vi "Get Recursive Dependency List.vi"(8 "error in":errorcluster, 11 "dependency paths":path[](array[path])) -> (0 "error out":errorcluster, 2 "instr containing":path[](array[path]), 3 "array":path[](array[path]))   [LabVIEW 2021, in "Converter.lvlib"]
uses:
  Converter.lvlib
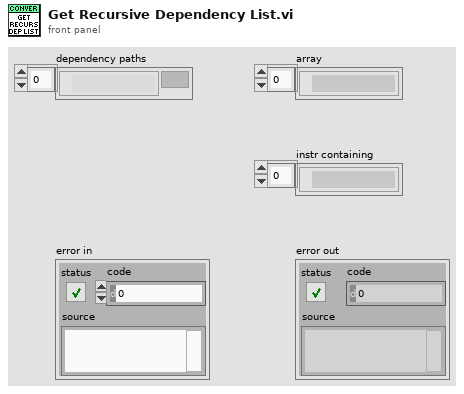
[diagram p1: front panel]
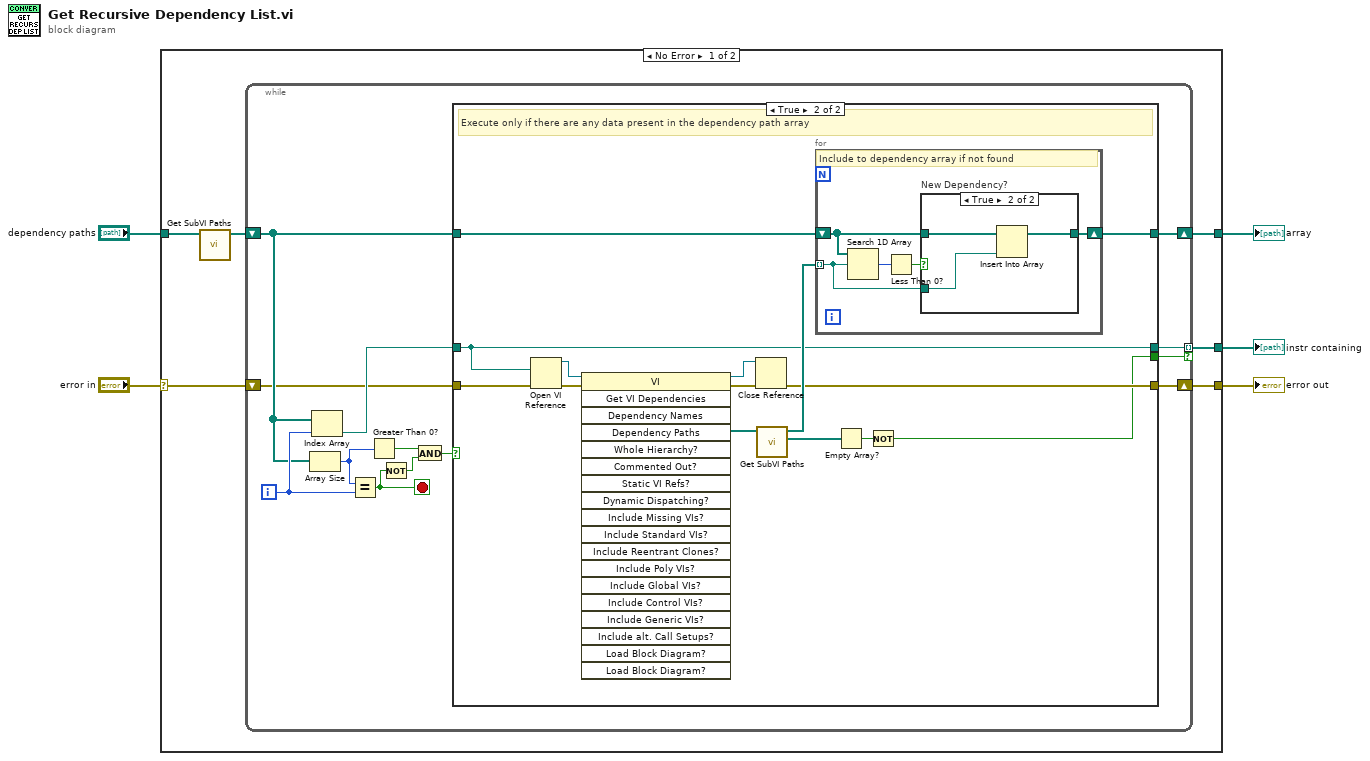
[diagram p0: block diagram]
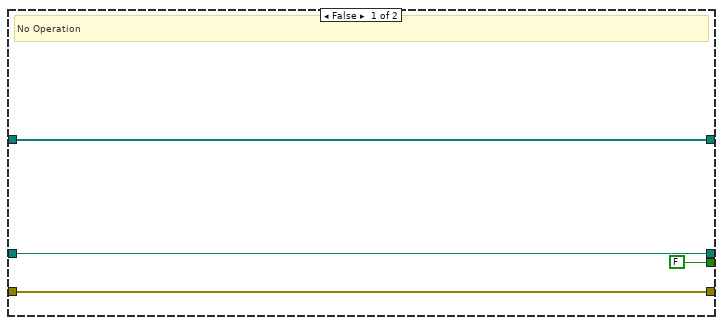
[diagram p2: hidden frame]
diagram:
  n1 = case shown="No Error" "error in" {
    selector: "error in" -> [w10 w52]
    tunnel: [w11 w52] -> w5
    tunnel: [w9 _] -> w3
    tunnel: "dependency paths" -> [w7 _]
    tunnel: [w6 _] -> w1
    frame No Error {
      n2 = call "Get SubVI Paths.vi"("dependency paths"=w7) -> ("actual dependencies[]"=w8:path[])  [unwired: 9 in, 1 out]
      n3 = while {
        shift-right: [w22] -> w9
        shift-left: w8 -> [w23]
        shift-right: [w19] -> w11
        shift-left: w10 -> [w20]
        tunnel: [w13] -> w6 mode=indexing if=w12
        i -> [w24]
        stop <- w17 stop-if-true
        n4 = Array Size(array=w23) -> (size(s)=w18:i32)
        n5 = Index Array(array=w23, index=w24) -> (element=w21:path)
        n6 = Equal?(x=w18, y=w24) -> (x = y?=w17:bool)
        n7 = Greater Than 0?(x=w18) -> (x > 0?=w15:bool)
        n8 = Not(x=w17) -> (.not. x?=w14:bool)
        n9 = And(x=w15, y=w14) -> (x .and. y?=w16:bool)
        n10 = case shown="True" w16 {
          tunnel: w23 -> [w27 w38]
          tunnel: [w27 w37] -> w22
          tunnel: w21 -> [w26 w32]
          tunnel: w20 -> [w28 w36]
          tunnel: [w28 w35] -> w19
          tunnel: [w26 w32] -> w13
          tunnel: [FALSE w31] -> w12
          frame False {
            # "No Operation"
          }
          frame True {
            # "Execute only if there are any data present in the dependency path array"
            n11 = Open VI Reference(vi path=w32, error in (no error)=w36) -> (vi reference=w41:refnum<vi>, error out=w42:errorcluster)  [unwired: 4 in]
            n12 = invoke class="VI" method="Get VI Dependencies"(reference=w41, error in=w42) -> (reference out=w30:refnum<vi>, error out=w29:errorcluster, "Dependency Paths"=w40:path[])  [unwired: 17 in, 16 out]
            n13 = Close Reference(reference=w30, error in (no error)=w29) -> (error out=w35:errorcluster)
            n14 = call "Get SubVI Paths.vi"("dependency paths"=w40) -> ("driver vis"=w34:path[], "actual dependencies[]"=w39:path[])  [unwired: 9 in]
            n15 = for {
              tunnel: w39 -> [w44] mode=indexing
              shift-right: [w43] -> w37
              shift-left: w38 -> [w45]
              # "Include to dependency array if not found"
              n16 = Search 1D Array(1D array=w45, element=w44) -> (index of element=w47:i32)  [unwired: 1 in]
              n17 = Less Than 0?(x=w47) -> (x < 0?=w46:bool)
              n18 = case "New Dependency?" shown="True" w46 {
                tunnel: w45 -> [w48 w51]
                tunnel: w44 -> [_ w50]
                tunnel: [w48 w49] -> w43
                frame False {
                }
                frame True {
                  n19 = Insert Into Array(array=w51, new element=w50) -> (w49:path[])  [unwired: 1 in]
                }
              }
            }
            n20 = Empty Array?(array=w34) -> (empty?=w33:bool)
            n21 = Not(x=w33) -> (.not. x?=w31:bool)
          }
        }
      }
    }
    frame Error {
    }
  }
  "error out" <- w5
  "array" <- w3
  "instr containing" <- w1
